vi "solar_excel Worksheet Rename.vi"(8 "error in (no error)":errorcluster, 10 "New Worksheet Name":string, 11 "Excel Worksheet in":T1) -> (0 "error out":errorcluster, 3 "Excel Worksheet out":T1)   [LabVIEW 2018]
doc: "This renames a Worksheet."
uses:
  solar_excel_ctl Worksheet.ctl
  solar_excel_ctl TSV.ctl
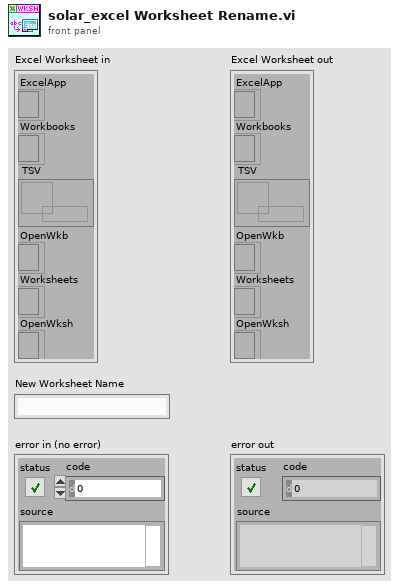
[diagram p1: front panel]
types:
  T1 = typedef "solar_excel_ctl Worksheet.ctl" = cluster{"ExcelApp":refnum<k7>, "Workbooks":refnum<k7>, "TSV":refnum<queue>, "OpenWkb":refnum<k7>, "Worksheets":refnum<k7>, "OpenWksh":refnum<k7>}
  T2 = typedef "solar_excel_ctl TSV.ctl" = cluster{"Path":path, "Dirty":bool, "ActiveSheet":u8, "Worksheets":string[], "Worksheet Cells":cluster{"Cells":string[][]}[]}
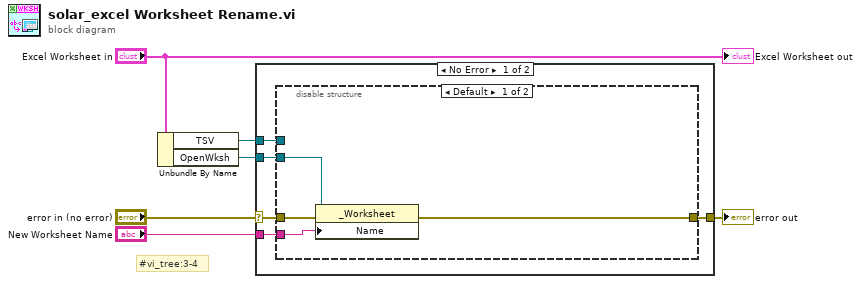
[diagram p0: block diagram]
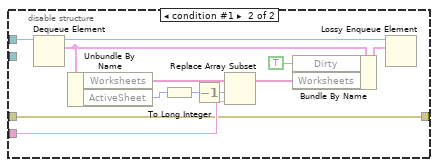
[diagram p2: hidden frame]
diagram:
  # "#vi_tree:3-4"
  n1 = Unbundle By Name("Excel Worksheet in") -> ("TSV"=w1:refnum<queue>, "OpenWksh"=w2:refnum<k7>)
  n2 = case shown="No Error" "error in (no error)" {
    selector: "error in (no error)" -> [w10 w28]
    tunnel: [w9 w28] -> w6
    tunnel: "New Worksheet Name" -> [w11 _]
    tunnel: w2 -> [w8 _]
    tunnel: w1 -> [w7 _]
    frame No Error {
      n3 = disable-structure shown="Default" {
        disable-tunnel: w11 -> [w15 w18]
        disable-tunnel: w10 -> [w14 w17]
        disable-tunnel: [w13 w17] -> w9
        disable-tunnel: w8 -> [w12 _]
        disable-tunnel: w7 -> [_ w27]
        frame condition #0 (active) {
          n4 = property class="_Worksheet"(reference=w12, error in=w14, "Name"=w15) -> (error out=w13:errorcluster)  [unwired: 1 out]
        }
        frame condition #1 {
          n5 = Dequeue Element(queue=w27) -> (queue out=w26:refnum<queue>, element=w25:T2)  [unwired: 2 in, 2 out]
          n6 = Unbundle By Name(w25) -> ("Worksheets"=w23:string[], "ActiveSheet"=w21:u8)
          n7 = To Long Integer(number=w21) -> (32bit integer=w20:i32)
          n8 = Decrement(x=w20) -> (x-1=w19:i32)
          n9 = Replace Array Subset(array=w23, new element=w18, index=w19) -> (w22:string[])
          n10 = Bundle By Name(cluster=w25, "Dirty"=TRUE, "Worksheets"=w22) -> (w24:T2)
          n11 = Lossy Enqueue Element(queue=w26, element=w24) -> ()  [unwired: 1 in, 4 out]
        }
      }
    }
    frame Error {
    }
  }
  "error out" <- w6
  "Excel Worksheet out" <- "Excel Worksheet in"
